vi "Populate Graphs.vi"(8 "error in (no error)":errorcluster, 9 "Array":dbl[][](array[numeric]), 10 "Red":refnum<vi>, 11 "Blue":refnum<vi>) -> (0 "error out":errorcluster)   [LabVIEW 2013, in "main.lvlib"]
uses:
  main.lvlib
panel:
  out "Waveform Graph":dbl[](graph)
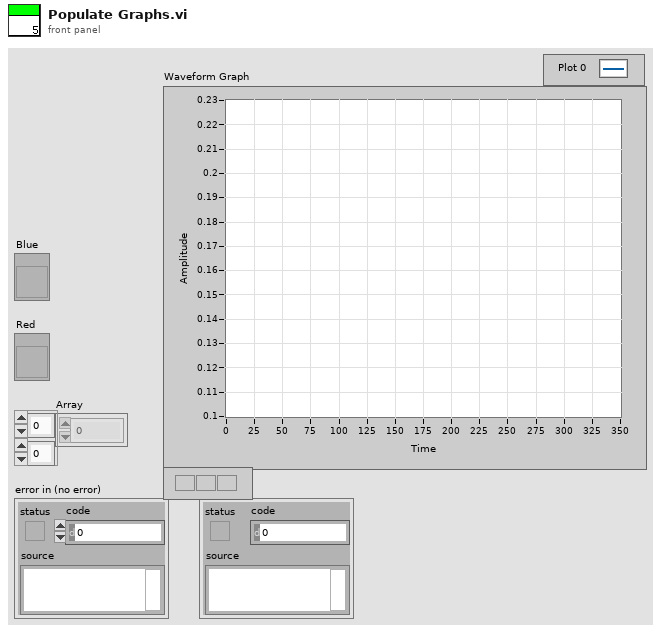
[diagram p1: front panel]
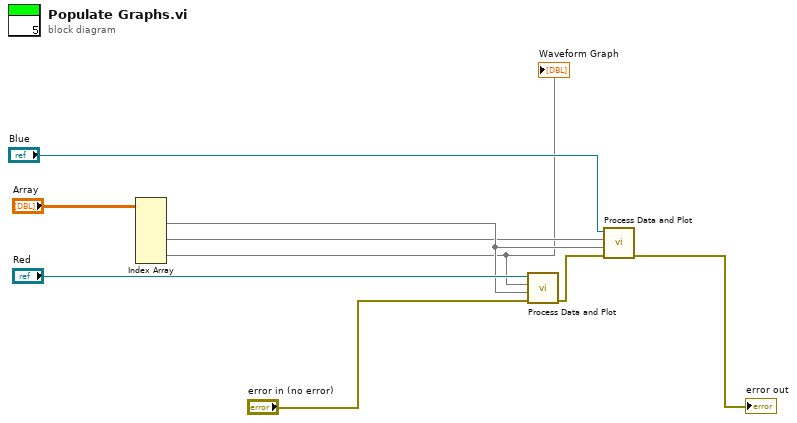
[diagram p0: block diagram]
diagram:
  n1 = Index Array(array="Array") -> (element #1=w3:dbl[], element #2=w2:dbl[], element #3=w1:dbl[])  [unwired: 6 in]
  "Waveform Graph" <- w1
  n2 = call "Process Data and Plot.vi"("error in (no error)"="error in (no error)", "Pressure"=w3, "Graph"=w1, "WaveformGraph in"="Red") -> ("error out"=w7:errorcluster)  [unwired: 7 in]
  n3 = call "Process Data and Plot.vi"("error in (no error)"=w7, "Pressure"=w3, "Graph"=w2, "WaveformGraph in"="Blue") -> ("error out"=→"error out":errorcluster)  [unwired: 7 in]
